vi "GetOPC_Stroke.vi"   [LabVIEW 2017]
uses:
  <vilib>/Utility/sysdir.llb/System Directory Type.ctl
  <vilib>/Utility/file.llb/Write Delimited Spreadsheet (string).vi
panel:
  # "Output file save to desktop !!!!"
types:
  T1 = typedef "System Directory Type.ctl" = i32
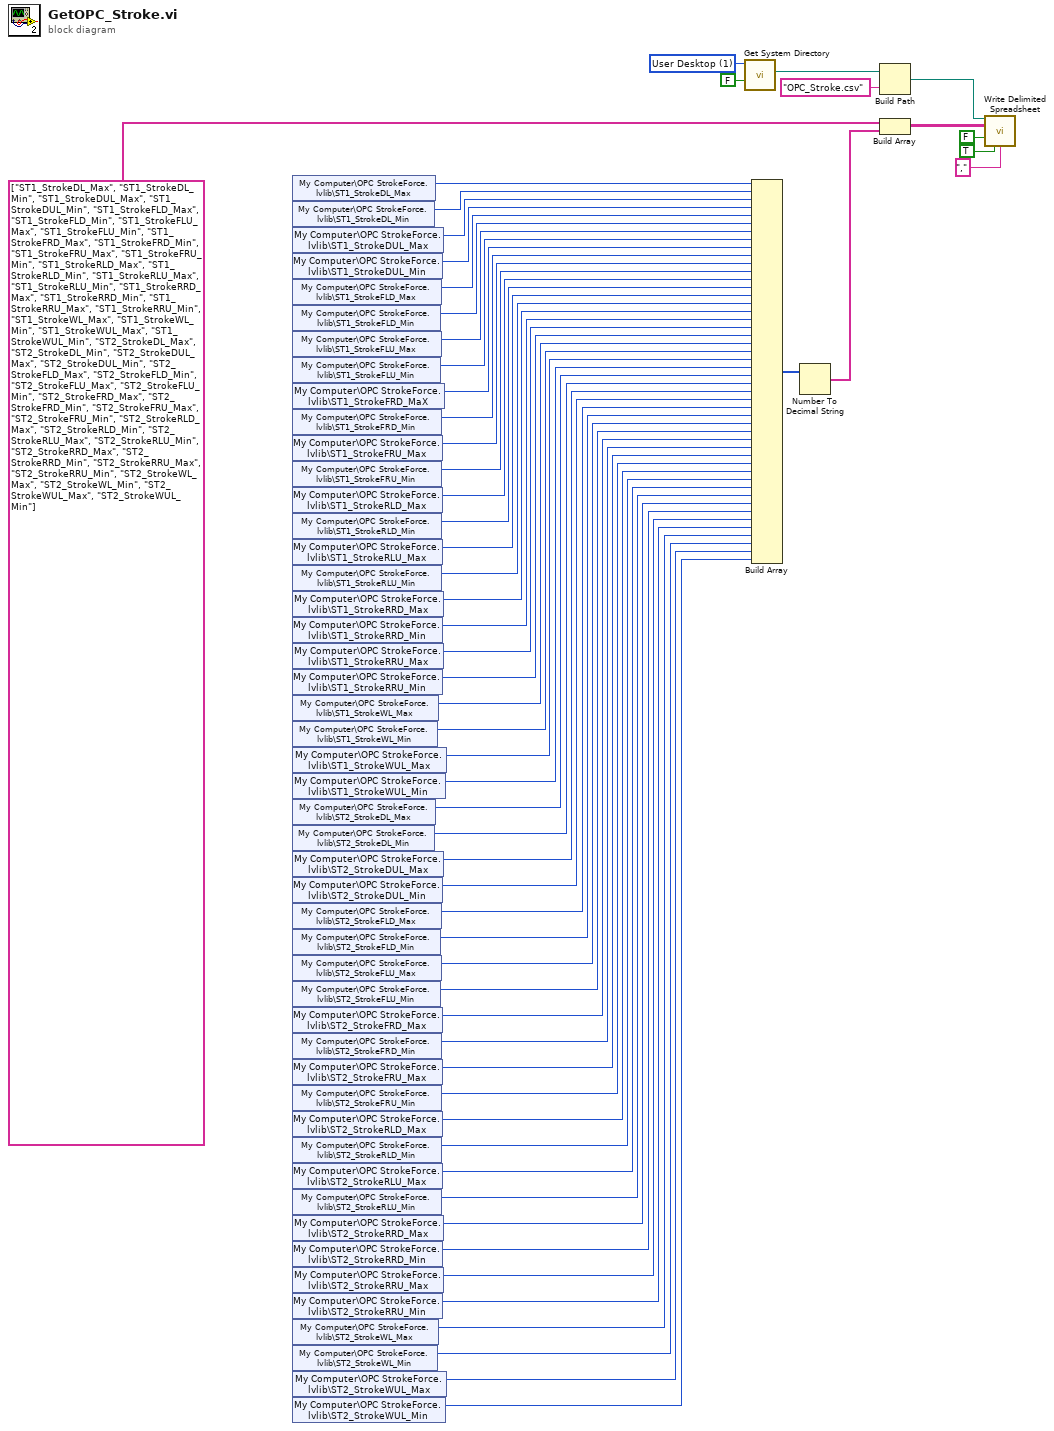
[diagram p0: block diagram]
diagram:
  w3 = T1 1 items=["User Home"=0, "User Desktop"=1, "User Documents"=2, "User Application Data"=3, "User Preferences"=4, "User Temporary"=5, "Public Documents"=6, "Public Application Data"=7, "Public Preferences"=8, "Public Cache"=13, "System Core Libraries"=9, "System Installed Libraries"=10, "Application Files"=11, "Boot Volume Root"=12] ("system directory type")
  n1 = shared-variable "My Computer\\OPC StrokeForce.lvlib\\ST1_StrokeDL_Max"() -> (w60:u16)  [unwired: 1 in, 1 out]
  n2 = shared-variable "My Computer\\OPC StrokeForce.lvlib\\ST1_StrokeDL_Min"() -> (w59:u16)  [unwired: 1 in, 1 out]
  n3 = shared-variable "My Computer\\OPC StrokeForce.lvlib\\ST1_StrokeDUL_Max"() -> (w58:u16)  [unwired: 1 in, 1 out]
  n4 = shared-variable "My Computer\\OPC StrokeForce.lvlib\\ST1_StrokeDUL_Min"() -> (w57:u16)  [unwired: 1 in, 1 out]
  n5 = shared-variable "My Computer\\OPC StrokeForce.lvlib\\ST1_StrokeFLD_Max"() -> (w56:u16)  [unwired: 1 in, 1 out]
  n6 = shared-variable "My Computer\\OPC StrokeForce.lvlib\\ST1_StrokeFLD_Min"() -> (w55:u16)  [unwired: 1 in, 1 out]
  n7 = shared-variable "My Computer\\OPC StrokeForce.lvlib\\ST1_StrokeFLU_Max"() -> (w54:u16)  [unwired: 1 in, 1 out]
  n8 = shared-variable "My Computer\\OPC StrokeForce.lvlib\\ST1_StrokeFLU_Min"() -> (w53:u16)  [unwired: 1 in, 1 out]
  n9 = shared-variable "My Computer\\OPC StrokeForce.lvlib\\ST1_StrokeFRD_MaX"() -> (w52:u16)  [unwired: 1 in, 1 out]
  n10 = shared-variable "My Computer\\OPC StrokeForce.lvlib\\ST1_StrokeFRD_Min"() -> (w51:u16)  [unwired: 1 in, 1 out]
  n11 = shared-variable "My Computer\\OPC StrokeForce.lvlib\\ST1_StrokeFRU_Max"() -> (w50:u16)  [unwired: 1 in, 1 out]
  n12 = shared-variable "My Computer\\OPC StrokeForce.lvlib\\ST1_StrokeFRU_Min"() -> (w49:u16)  [unwired: 1 in, 1 out]
  n13 = shared-variable "My Computer\\OPC StrokeForce.lvlib\\ST1_StrokeRLD_Max"() -> (w48:u16)  [unwired: 1 in, 1 out]
  n14 = shared-variable "My Computer\\OPC StrokeForce.lvlib\\ST1_StrokeRLD_Min"() -> (w47:u16)  [unwired: 1 in, 1 out]
  n15 = shared-variable "My Computer\\OPC StrokeForce.lvlib\\ST1_StrokeRLU_Max"() -> (w46:u16)  [unwired: 1 in, 1 out]
  n16 = shared-variable "My Computer\\OPC StrokeForce.lvlib\\ST1_StrokeRLU_Min"() -> (w45:u16)  [unwired: 1 in, 1 out]
  n17 = shared-variable "My Computer\\OPC StrokeForce.lvlib\\ST1_StrokeRRD_Max"() -> (w44:u16)  [unwired: 1 in, 1 out]
  n18 = shared-variable "My Computer\\OPC StrokeForce.lvlib\\ST1_StrokeRRD_Min"() -> (w43:u16)  [unwired: 1 in, 1 out]
  n19 = shared-variable "My Computer\\OPC StrokeForce.lvlib\\ST1_StrokeRRU_Max"() -> (w42:u16)  [unwired: 1 in, 1 out]
  n20 = shared-variable "My Computer\\OPC StrokeForce.lvlib\\ST1_StrokeRRU_Min"() -> (w41:u16)  [unwired: 1 in, 1 out]
  n21 = shared-variable "My Computer\\OPC StrokeForce.lvlib\\ST1_StrokeWL_Max"() -> (w40:u16)  [unwired: 1 in, 1 out]
  n22 = shared-variable "My Computer\\OPC StrokeForce.lvlib\\ST1_StrokeWL_Min"() -> (w39:u16)  [unwired: 1 in, 1 out]
  n23 = shared-variable "My Computer\\OPC StrokeForce.lvlib\\ST1_StrokeWUL_Max"() -> (w38:u16)  [unwired: 1 in, 1 out]
  n24 = shared-variable "My Computer\\OPC StrokeForce.lvlib\\ST1_StrokeWUL_Min"() -> (w37:u16)  [unwired: 1 in, 1 out]
  n25 = shared-variable "My Computer\\OPC StrokeForce.lvlib\\ST2_StrokeDL_Max"() -> (w36:u16)  [unwired: 1 in, 1 out]
  n26 = shared-variable "My Computer\\OPC StrokeForce.lvlib\\ST2_StrokeDL_Min"() -> (w35:u16)  [unwired: 1 in, 1 out]
  n27 = shared-variable "My Computer\\OPC StrokeForce.lvlib\\ST2_StrokeDUL_Max"() -> (w34:u16)  [unwired: 1 in, 1 out]
  n28 = shared-variable "My Computer\\OPC StrokeForce.lvlib\\ST2_StrokeDUL_Min"() -> (w33:u16)  [unwired: 1 in, 1 out]
  n29 = shared-variable "My Computer\\OPC StrokeForce.lvlib\\ST2_StrokeFLD_Max"() -> (w32:u16)  [unwired: 1 in, 1 out]
  n30 = shared-variable "My Computer\\OPC StrokeForce.lvlib\\ST2_StrokeFLD_Min"() -> (w31:u16)  [unwired: 1 in, 1 out]
  n31 = shared-variable "My Computer\\OPC StrokeForce.lvlib\\ST2_StrokeFLU_Max"() -> (w30:u16)  [unwired: 1 in, 1 out]
  n32 = shared-variable "My Computer\\OPC StrokeForce.lvlib\\ST2_StrokeFLU_Min"() -> (w29:u16)  [unwired: 1 in, 1 out]
  n33 = shared-variable "My Computer\\OPC StrokeForce.lvlib\\ST2_StrokeFRD_Max"() -> (w28:u16)  [unwired: 1 in, 1 out]
  n34 = shared-variable "My Computer\\OPC StrokeForce.lvlib\\ST2_StrokeFRD_Min"() -> (w27:u16)  [unwired: 1 in, 1 out]
  n35 = shared-variable "My Computer\\OPC StrokeForce.lvlib\\ST2_StrokeFRU_Max"() -> (w26:u16)  [unwired: 1 in, 1 out]
  n36 = shared-variable "My Computer\\OPC StrokeForce.lvlib\\ST2_StrokeFRU_Min"() -> (w25:u16)  [unwired: 1 in, 1 out]
  n37 = shared-variable "My Computer\\OPC StrokeForce.lvlib\\ST2_StrokeRLD_Max"() -> (w24:u16)  [unwired: 1 in, 1 out]
  n38 = shared-variable "My Computer\\OPC StrokeForce.lvlib\\ST2_StrokeRLD_Min"() -> (w23:u16)  [unwired: 1 in, 1 out]
  n39 = shared-variable "My Computer\\OPC StrokeForce.lvlib\\ST2_StrokeRLU_Max"() -> (w22:u16)  [unwired: 1 in, 1 out]
  n40 = shared-variable "My Computer\\OPC StrokeForce.lvlib\\ST2_StrokeRLU_Min"() -> (w21:u16)  [unwired: 1 in, 1 out]
  n41 = shared-variable "My Computer\\OPC StrokeForce.lvlib\\ST2_StrokeRRD_Max"() -> (w20:u16)  [unwired: 1 in, 1 out]
  n42 = shared-variable "My Computer\\OPC StrokeForce.lvlib\\ST2_StrokeRRD_Min"() -> (w19:u16)  [unwired: 1 in, 1 out]
  n43 = shared-variable "My Computer\\OPC StrokeForce.lvlib\\ST2_StrokeRRU_Max"() -> (w18:u16)  [unwired: 1 in, 1 out]
  n44 = shared-variable "My Computer\\OPC StrokeForce.lvlib\\ST2_StrokeRRU_Min"() -> (w17:u16)  [unwired: 1 in, 1 out]
  n45 = shared-variable "My Computer\\OPC StrokeForce.lvlib\\ST2_StrokeWL_Max"() -> (w16:u16)  [unwired: 1 in, 1 out]
  n46 = shared-variable "My Computer\\OPC StrokeForce.lvlib\\ST2_StrokeWL_Min"() -> (w15:u16)  [unwired: 1 in, 1 out]
  n47 = shared-variable "My Computer\\OPC StrokeForce.lvlib\\ST2_StrokeWUL_Max"() -> (w14:u16)  [unwired: 1 in, 1 out]
  n48 = shared-variable "My Computer\\OPC StrokeForce.lvlib\\ST2_StrokeWUL_Min"() -> (w13:u16)  [unwired: 1 in, 1 out]
  n49 = call <vilib>:"Get System Directory.vi"("create directory if not found? (F)"=FALSE, "system directory type"=w3) -> ("system directory"=w2:path)  [unwired: 9 in]
  n50 = Build Array(w60, w59, w58, w57, w56, w55, w54, w53, w52, w51, w50, w49, w48, w47, w46, w45, w44, w43, w42, w41, w40, w39, w38, w37, w36, w35, w34, w33, w32, w31, w30, w29, w28, w27, w26, w25, w24, w23, w22, w21, w20, w19, w18, w17, w16, w15, w14, w13) -> (w11:u16[])
  n51 = Number To Decimal String(number=w11) -> (decimal integer string=w10:string[])  [unwired: 1 in]
  n52 = Build Path(base path=w2, name or relative path="OPC_Stroke.csv") -> (appended path=w5:path)
  n53 = Build Array(string[] ["ST1_StrokeDL_Max", "ST1_StrokeDL_Min", "ST1_StrokeDUL_Max", "ST1_StrokeDUL_Min", "ST1_StrokeFLD_Max", "ST1_StrokeFLD_Min", "ST1_StrokeFLU_Max", "ST1_StrokeFLU_Min", "ST1_StrokeFRD_Max", "ST1_StrokeFRD_Min", "ST1_StrokeFRU_Max", "ST1_StrokeFRU_Min", "ST1_StrokeRLD_Max", "ST1_StrokeRLD_Min", "ST1_StrokeRLU_Max", "ST1_StrokeRLU_Min", "ST1_StrokeRRD_Max", "ST1_StrokeRRD_Min", "ST1_StrokeRRU_Max", "ST1_StrokeRRU_Min", "ST1_StrokeWL_Max", "ST1_StrokeWL_Min", "ST1_StrokeWUL_Max", "ST1_StrokeWUL_Min", "ST2_StrokeDL_Max", "ST2_StrokeDL_Min", "ST2_StrokeDUL_Max", "ST2_StrokeDUL_Min", "ST2_StrokeFLD_Max", "ST2_StrokeFLD_Min", "ST2_StrokeFLU_Max", "ST2_StrokeFLU_Min", "ST2_StrokeFRD_Max", "ST2_StrokeFRD_Min", "ST2_StrokeFRU_Max", "ST2_StrokeFRU_Min", "ST2_StrokeRLD_Max", "ST2_StrokeRLD_Min", "ST2_StrokeRLU_Max", "ST2_StrokeRLU_Min", "ST2_StrokeRRD_Max", "ST2_StrokeRRD_Min", "ST2_StrokeRRU_Max", "ST2_StrokeRRU_Min", "ST2_StrokeWL_Max", "ST2_StrokeWL_Min", "ST2_StrokeWUL_Max", "ST2_StrokeWUL_Min"], w10) -> (w9:string[][])
  n54 = call-poly <vilib>:"Write Delimited Spreadsheet.vi"("file path (dialog if empty)"=w5, "2D data"=w9, "append to file? (new file:F)"=FALSE, "transpose? (no:F)"=TRUE, "delimiter (\\t)"="," ("delimiter (\\t)")) -> ()  [unwired: 9 in, 2 out]
